vi "Read Port.vi"(8 "error in (no error)":errorcluster, 9 "Timeout":i16, 11 "TestMPU in":refnum<class "TestMPU.lvclass">) -> (0 "error out":errorcluster, 1 "Timeouted":bool, 2 "Data":u8, 3 "TestMPU out":refnum<class "TestMPU.lvclass">)   [LabVIEW 2018, in "TestMPU.lvclass"]
uses:
  TestMPU.lvclass
  TestMPU.lvclass/TestMPU.ctl
  <vilib>/rvi/DataTransferAndStorage/Container/Common/niFpgaContainerExecOnDevCompGetState.vi
  <vilib>/rvi/Emulation/niFpgaEmulationIsFPGAContextNoSignature.vi
  <vilib>/rvi/Emulation/niFpgaSctlEmulationGetInTimedLoop.vi
  <vilib>/rvi/errors/niFpgaSetErrorForExecOnDevCompSimple.vi
  <vilib>/rvi/eio/common/nirviEmuReportErrorAndStop.vi
  <vilib>/rvi/DataTransferAndStorage/Container/Common/niFpgaContainerGetUniqueNameForEmu.vi
  <vilib>/rvi/FIFO/Fifo_Resource/nirvififoEmulationSetSize.vi
  <vilib>/rvi/FIFO/Fifo_Resource/nirviFifoEmulationQueueMgr.vi
  <instcachedir>/0/nirviFifoEmulationQueueMgr_E5CAEC123FF24DC58D834DCA3CDAA9B5.lvgen/nirviFifoEmulationQueueMgr_E5CAEC123FF24DC58D834DCA3CDAA9B5_001.vi
  <vilib>/rvi/FIFO/Fifo_Resource/nirvififoEmulationDetermineInputValidOut.vi
  <vilib>/rvi/FIFO/Fifo_Resource/nirvififoEmulationCreateLock.vi
  <vilib>/rvi/Emulation/niFpgaProcessEmulError.vi
  <vilib>/rvi/FIFO/Fifo_Resource/nirvififoEmulationObtainLock.vi
  <vilib>/rvi/FIFO/Fifo_Resource/nirvififoEmulationReleaseLock.vi
  <vilib>/rvi/occurrence/nirviWaitOnOccurrenceBase.vi
  <vilib>/rvi/errors/nirviReportUnexpectedCaseInternalError.vi
  <vilib>/rvi/errors/nirviReportUnexpectedCaseInternalError (U32).vi
  <vilib>/Utility/error.llb/Clear Errors.vi
  <vilib>/rvi/interface/RandomDataEmulation/niFpgaRandomDataHandleErrors.vi
  <vilib>/rvi/DataTransferAndStorage/Container/XNode/niFpgaContainer.xnode
  <vilib>/rvi/FIFO/Fifo_Resource/niFpgaFifoEmulationRefIn.vi
  src/MPU.lvclass
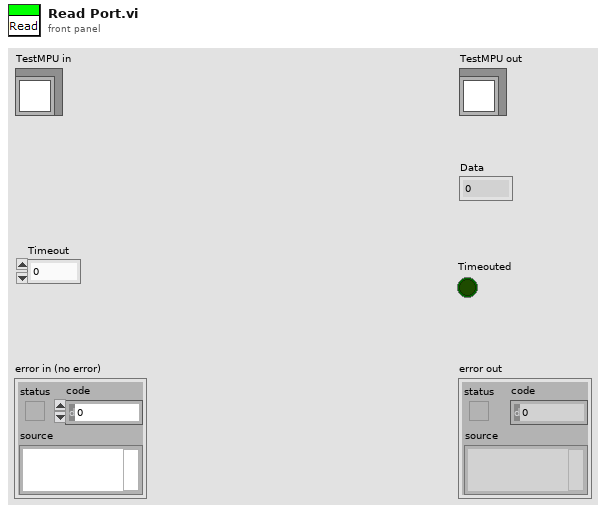
[diagram p1: front panel]
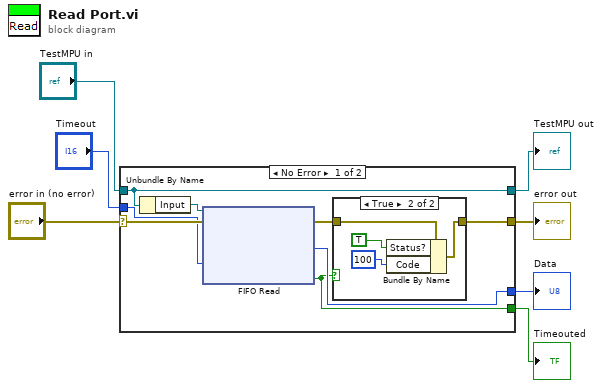
[diagram p0: block diagram]
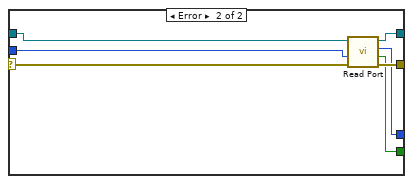
[diagram p3: hidden frame]
diagram:
  n1 = case shown="No Error" "error in (no error)" {
    selector: "error in (no error)" -> [w13 w22]
    tunnel: [w8 w27] -> w7
    tunnel: [w10 w26] -> w6
    tunnel: [w11 w25] -> w5
    tunnel: "Timeout" -> [w12 w24]
    tunnel: "TestMPU in" -> [w15 w23]
    tunnel: [w15 w21] -> w1
    frame No Error {
      n2 = Unbundle By Name(w15) -> ("Input"=w14:refnum<k21>)
      n3 = xnode "FIFO Read"("Timeout"=w12, "error in (no error)"=w13, "FIFO In"=w14) -> ("Element"=w11:u8, "Timed Out?"=w10:bool, "error out"=w9:errorcluster)  [unwired: 1 out]
      n4 = case shown="True" w10 {
        tunnel: [w16 w19] -> w8
        tunnel: w9 -> [w16 w20]
        frame False {
        }
        frame True {
          n5 = Bundle By Name(cluster=w20, "Status?"=TRUE, "Code"=100) -> (w19:errorcluster)
        }
      }
    }
    frame Error {
      n6 = call-parent "Read Port.vi"("error in (no error)"=w22, "Timeout"=w24, "MPU in"=w23) -> ("error out"=w27:errorcluster, "Timeouted"=w26:bool, "Data"=w25:u8, "MPU out"=w21:refnum<class "TestMPU.lvclass">)  [unwired: 5 in]
    }
  }
  "error out" <- w7
  "TestMPU out" <- w1
  "Data" <- w5
  "Timeouted" <- w6
